vi "ReadXLSConfig.vi"(8 "error in":errorcluster caption="错误输入", 9 "pagename":string, 10 "XLSName":string, 11 "PathIn":path) -> (0 "error out":errorcluster caption="错误输出", 3 "Data":string[][](array[string]))   [LabVIEW 2013]
uses:
  <vilib>/Utility/NIReport.llb/NI_report.lvclass
  <vilib>/addons/_office/excel.llb/Excel Get Data ([str]).vi
  <vilib>/addons/_office/NI_ReportGenerationToolkit.lvlib
  <vilib>/Utility/NIReport.llb/Excel/NI_Excel.lvclass
panel:
  out "ConfigPath":string="C:\\Users\\dell\\Desktop\\ExcelReport.vi"
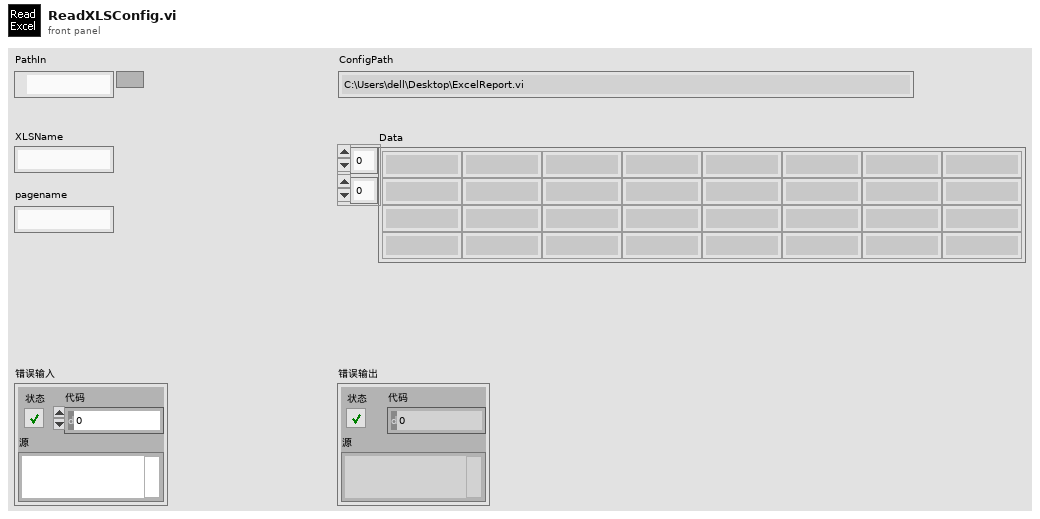
[diagram p1: front panel]
types:
  T1 = enum16{"maximized", "minimized", "normal", "no change"}
  T2 = enum16{"Standard Report", "HTML", "Word", "Excel"}
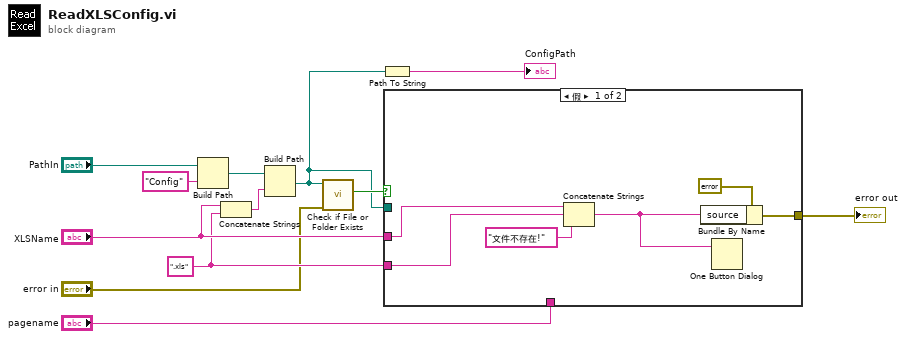
[diagram p0: block diagram]
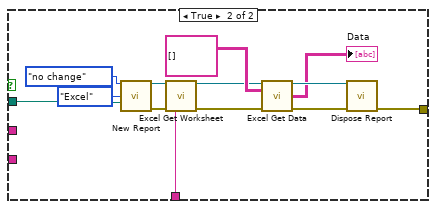
[diagram p2: hidden frame]
diagram:
  w8 = ".xls" ("字符串")
  n1 = Build Path(base path="PathIn", name or relative path="Config" ("名称或相对路径")) -> (appended path=w10:path)
  n2 = Concatenate Strings("XLSName", w8) -> (w7:string)
  n3 = Build Path(base path=w10, name or relative path=w7) -> (appended path=w2:path)
  n4 = call <vilib>:"Check if File or Folder Exists.vi"("error in (no error)"="error in", "path"=w2) -> ("file or folder exists?"=w5:bool)  [unwired: 7 in, 2 out]
  n5 = Path To String(path=w2) -> (string=→"ConfigPath":string)
  n6 = case shown="假" w5 {
    tunnel: [w18 w26] -> w4
    tunnel: "XLSName" -> [w17 _]
    tunnel: w8 -> [w16 _]
    tunnel: w2 -> [_ w21]
    tunnel: "pagename" -> [_ w20]
    frame False {
      n7 = Concatenate Strings(w17, w16, "文件不存在!" ("消息")) -> (w14:string)
      n8 = Bundle By Name(cluster=errorcluster {"status"=TRUE, "code"=5000, "source"=""} ("error in 1 (no error)"), "source"=w14) -> (w18:errorcluster)
      n9 = One Button Dialog(message=w14) -> ()  [unwired: 1 in, 1 out]
    }
    frame True {
      n10 = call <vilib>:"New Report.vi"("window state (normal)"=T1."no change", "report type"=T2."Excel", "template (empty)"=w21) -> ("report out"=w25:refnum<class "NI_report.lvclass">, "error out"=w22:errorcluster)  [unwired: 3 in, 8 out]
      n11 = call <vilib>:"Excel Get Worksheet.vi"("report in"=w25, "error in (no error)"=w22, "name (\"\")"=w20) -> ("report out"=w24:refnum<class "NI_report.lvclass">, "error out"=w23:errorcluster)  [unwired: 11 in]
      n12 = call-poly <vilib>:"Excel Get Data.vi"("report in"=w24, "data type"=string[][] [], "error in (no error)"=w23) -> ("report out"=w28:refnum<class "NI_report.lvclass">, "data"=→"Data":string[][], "error out"=w27:errorcluster)  [unwired: 10 in]
      n13 = call-dynamic "Dispose Report.vi"("report in"=w28, "error in (no error)"=w27) -> ("error out"=w26:errorcluster)  [unwired: 3 in, 10 out]
    }
  }
  "error out" <- w4
